vi "DifferentialVelocityVoltage SetControl.vi"(0 "DeviceReference":T1, 1 "StopSendingOtherRequests":bool=TRUE, 2 "TargetVelocity":dbl, 3 "DifferentialPosition":dbl, 4 "EnableFOC":bool=TRUE, 5 "TargetSlot":i32, 6 "DifferentialSlot":i32=1, 7 "error in":errorcluster, 8 "OverrideBrakeDurNeutral":bool, 9 "LimitForwardMotion":bool, 10 "LimitReverseMotion":bool, 11 "IgnoreHardwareLimits":bool, 12 "UseTimesync":bool, 18 "Update Frequency (Hz)":dbl=100.0) -> (20 "DeviceReference Out":T1, 27 "error out":errorcluster)   [LabVIEW 2023]
doc: "Request PID to target velocity with a differential position setpoint.\nThis control mode will set the motor's velocity setpoint to the velocity specified by the user. It will also set the motor's differential position setpoint to the specified position."
uses:
  Users/test.DESKTOP-CORY/Documents/PhoenixProLabVIEWGeneration/CopyDown/DeviceReference.ctl
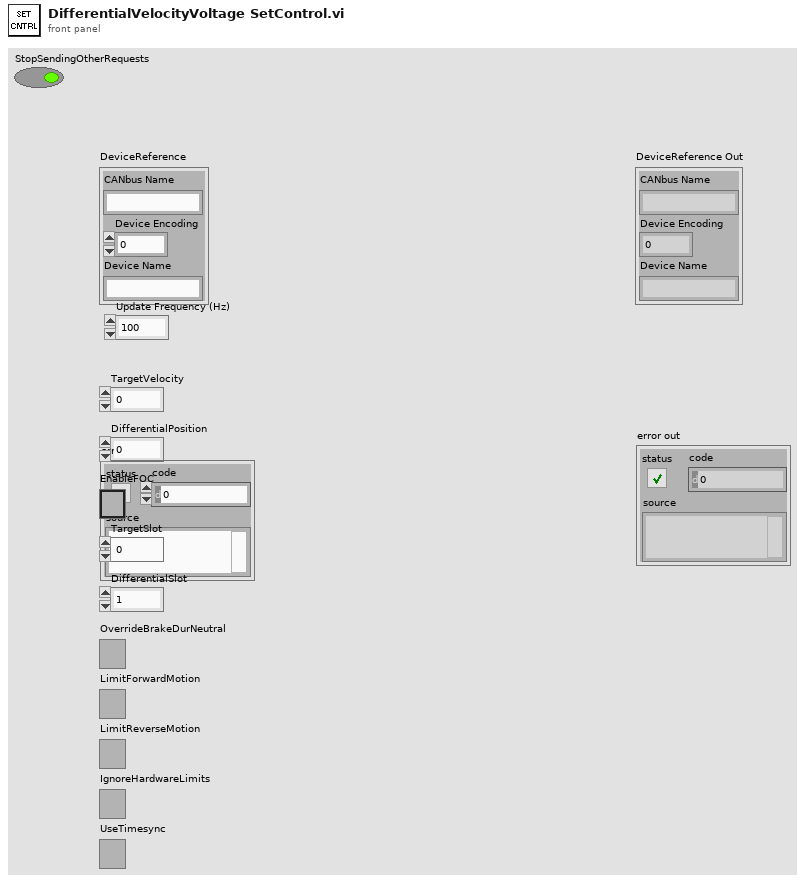
[diagram p1: front panel]
types:
  T1 = typedef "DeviceReference.ctl" = cluster{"CANbus Name":string, "Device Encoding":u32, "Device Name":string}
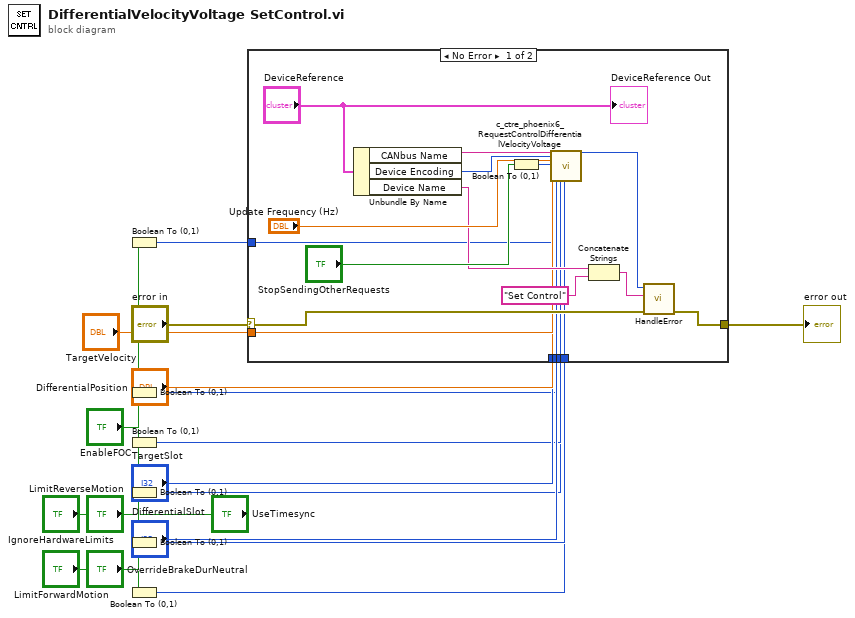
[diagram p0: block diagram]
diagram:
  n1 = Boolean To (0,1)(Boolean="EnableFOC") -> (0, 1=w13:i16)
  n2 = Boolean To (0,1)(Boolean="OverrideBrakeDurNeutral") -> (0, 1=w9:i16)
  n3 = Boolean To (0,1)(Boolean="LimitForwardMotion") -> (0, 1=w7:i16)
  n4 = Boolean To (0,1)(Boolean="LimitReverseMotion") -> (0, 1=w5:i16)
  n5 = Boolean To (0,1)(Boolean="IgnoreHardwareLimits") -> (0, 1=w3:i16)
  n6 = Boolean To (0,1)(Boolean="UseTimesync") -> (0, 1=w1:i16)
  n7 = case shown="No Error" "error in" {
    selector: "error in" -> [w33 w41]
    tunnel: [w32 w41] -> w17
    tunnel: "TargetVelocity" -> [w28 _]
    tunnel: "DifferentialPosition" -> [w27 _]
    tunnel: w13 -> [w26 _]
    tunnel: "TargetSlot" -> [w25 _]
    tunnel: "DifferentialSlot" -> [w24 _]
    tunnel: w9 -> [w23 _]
    tunnel: w7 -> [w22 _]
    tunnel: w5 -> [w21 _]
    tunnel: w3 -> [w20 _]
    tunnel: w1 -> [w19 _]
    frame No Error {
      n8 = Unbundle By Name("DeviceReference") -> ("CANbus Name"=w39:string, "Device Encoding"=w38:u32, "Device Name"=w31:string)
      n9 = Boolean To (0,1)(Boolean="StopSendingOtherRequests") -> (0, 1=w35:i16)
      n10 = call <vilib>:"c_ctre_phoenix6_RequestControlDifferentialVelocityVoltage.vi"("String 2"=w39, "Numeric 2"=w38, "Numeric 3"="Update Frequency (Hz)", "Numeric 4"=w35, "Numeric 5"=w28, "Numeric 6"=w27, "Numeric 7"=w26, "Numeric 8"=w25, "Numeric 9"=w24, "Numeric 10"=w23, "Numeric 11"=w22, "Numeric 12"=w21, "Numeric 13"=w20, 13:w19) -> ("Numeric"=w34:i32)  [unwired: 12 in, 1 out]
      n11 = Concatenate Strings(w31, "Set Control" ("origin")) -> (w29:string)
      n12 = call "HandleError.vi"("error in"=w33, "origin"=w29, "Status"=w34) -> ("error out"=w32:errorcluster)  [unwired: 8 in]
      "DeviceReference Out" <- "DeviceReference"
    }
    frame Error {
    }
  }
  "error out" <- w17
